vi "Create NI 9224.vi"(8 "error in":errorcluster, 10 "conversion time":T2, 11 "channel settings":T1[](array[typedef])) -> (0 "error out":errorcluster, 3 "NI 9224 out":refnum<class "NI 9224.lvclass">)   [LabVIEW 2020, in "Scan Engine Scripting.lvlib" / "NI 9224.lvclass"]
doc: "Creates and configures an instance of a NI-9224 analog input module that can be used to set a slot in a Scan Engine custom device chassis."
uses:
  NI 9224.lvclass
  Utility/Shared Properties/Conversion Time.ctl
  Mode Classes/Controls/analog channel settings.ctl
  Mode Classes/Analog Input Mode/Analog Input Vrms Mode/Analog Input Mode.lvclass
  C:/jenkins/workspace/ercat-custom-device_release_20.4/Custom Device Source/Scripting/Modules/Mode Classes/Mode/Mode.lvclass
  NI 9224.lvclass/NI 9224.ctl
  ef383861-b0bd-41a9-9063-6c2dc32b700d.vi
  Scan Engine Scripting.lvlib
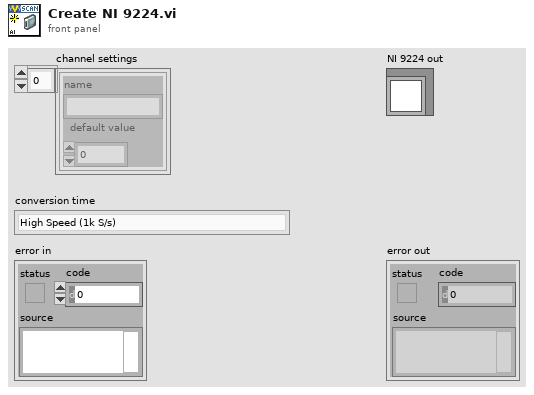
[diagram p1: front panel]
types:
  T1 = typedef "Scan Engine Scripting.lvlib/analog channel settings.ctl" = cluster{"name":string, "default value":dbl}
  T2 = typedef "Scan Engine Scripting.lvlib/Conversion Time.ctl" = enum16{"High Speed (1k S/s)", "Medium Speed (100 S/s)", "Medium Resolution (50/60Hz Rejection - 12 S/s)", "High Resolution (50/60Hz Rejection - 2 S/s)"}
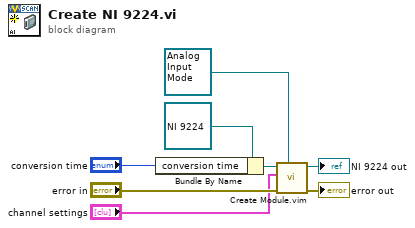
[diagram p0: block diagram]
diagram:
  n1 = Bundle By Name(cluster=refnum<class "NI 9224.lvclass"> refnum ("NI 9224 in"), "conversion time"="conversion time") -> (w4:refnum<class "NI 9224.lvclass">)
  n2 = call "Create Module.vim"("mode"=refnum<class "Analog Input Mode.lvclass"> refnum ("Scan Engine Scripting.lvlib:Analog Input Mode.lvclass"), "error in"="error in", "channel settings"="channel settings", "module in"=w4) -> ("error out"=→"error out":errorcluster, "module out"=→"NI 9224 out":refnum<class "NI 9224.lvclass">)  [unwired: 6 in]
